vi "svc_Unit Label Lexical Class.vi"(7 "unit label":string) -> (3 "letters only?":bool)   [LabVIEW 2017]
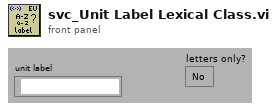
[diagram p1: front panel]
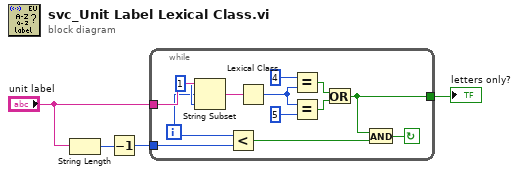
[diagram p0: block diagram]
diagram:
  n1 = String Length(string="unit label") -> (length=w1:i32)
  n2 = Decrement(x=w1) -> (x-1=w2:i32)
  n3 = while {
    tunnel: [w5] -> w3
    tunnel: w2 -> [w8]
    tunnel: "unit label" -> [w17]
    i -> [w9]
    stop <- w6 continue-if-true
    n4 = String Subset(string=w17, offset (0)=w9, length (rest)=1 ("length")) -> (substring=w15:string)
    n5 = Less?(x=w9, y=w8) -> (x < y?=w7:bool)
    n6 = Lexical Class(1:w15) -> (0:w14:i16)
    n7 = Equal?(x=i16 4, y=w14) -> (x = y?=w11:bool)
    n8 = Equal?(x=w14, y=i16 5) -> (x = y?=w10:bool)
    n9 = Or(x=w11, y=w10) -> (x .or. y?=w5:bool)
    n10 = And(x=w5, y=w7) -> (x .and. y?=w6:bool)
  }
  "letters only?" <- w3
